vi "waitForIdleAndPrintTaskInfo.vi"(8 "error in (no error)":errorcluster, 9 "Timeout, ms (-1)":i32=-1, 10 "wait for ApplicationState (Idle)":i32(ring)=1448165379 items=["NotRunning"=1448165376, "Starting"=1448165377, "Dying"=1448165378, "Idle"=1448165379, "WorkInProgress"=1448165380], 11 "VGS_RemoteControlClient in":refnum<class "VGS_RemoteControlClient.lvclass">) -> (0 "error out":errorcluster, 3 "VGS_RemoteControlClient out":refnum<class "VGS_RemoteControlClient.lvclass">)   [LabVIEW 2022 SP3, in "LV_VGS.lvlib" / "VGS_RemoteControlClient.lvclass"]
uses:
  VGS_RemoteControlClient.lvclass
panel:
  # "< do not change default, please"
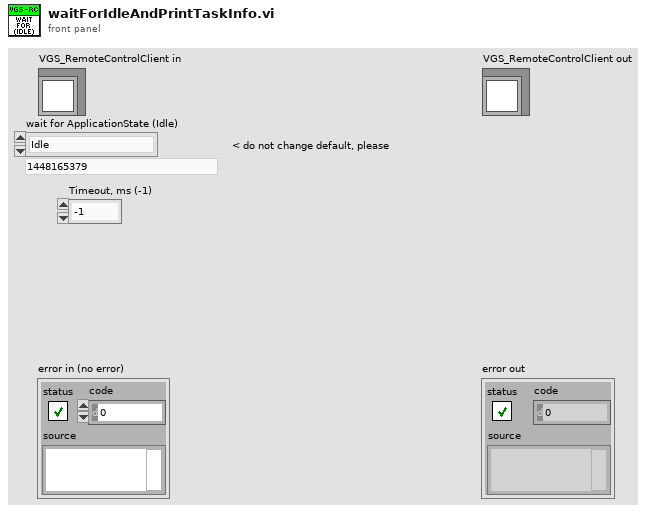
[diagram p1: front panel]
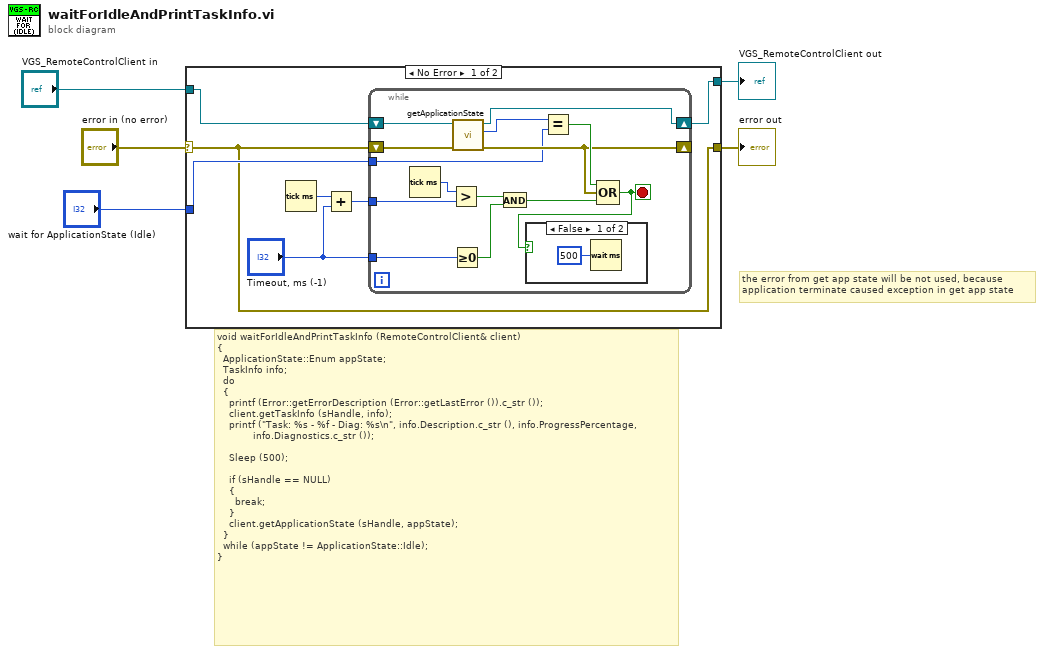
[diagram p0: block diagram]
diagram:
  # "the error from get app state will be not used, because\napplication terminate caused exception in get app state"
  # "void waitForIdleAndPrintTaskInfo (RemoteControlClient& client)\n{\n  ApplicationState::Enum appState;\n  TaskInfo info;\n  do\n  {\n    printf (Error::getErrorDescription (Error::getLastError ()).c_str ());\n    client.getTaskInfo (sHandle, info);\n    printf (\"Task: %s - %f - Diag: %s\\n\", info.Description.c_str (), info.ProgressPercentage,\n            info.Diagnostics.c_str ());\n\n    Sleep (500);\n\n    if (sHandle == NULL)\n    {\n      break;\n    }\n    client.getApplicationState (sHandle, appState);\n  }\n  while (appState != ApplicationState::Idle);\n}"
  n1 = case shown="No Error" "error in (no error)" {
    selector: "error in (no error)" -> [w6 w29]
    tunnel: [w6 w29] -> w4
    tunnel: [w11 w28] -> w2
    tunnel: "VGS_RemoteControlClient in" -> [w12 w28]
    tunnel: "wait for ApplicationState (Idle)" -> [w7 _]
    frame No Error {
      n2 = Tick Count (ms)() -> (millisecond timer value=w10:u32)
      n3 = Add(x=w10, y="Timeout, ms (-1)") -> (x+y=w9:u32)
      n4 = while {
        shift-right: [w26] -> w11
        shift-left: w12 -> [w13]
        shift-right: [w23] -> _
        shift-left: w6 -> [w14]
        tunnel: w9 -> [w21]
        tunnel: "Timeout, ms (-1)" -> [w19]
        tunnel: w7 -> [w16]
        stop <- w15 stop-if-true
        n5 = Tick Count (ms)() -> (millisecond timer value=w22:u32)
        n6 = Greater?(x=w22, y=w21) -> (0:w20:bool)
        n7 = Greater Or Equal To 0?(x=w19) -> (x >= 0?=w18:bool)
        n8 = call "getApplicationState.vi"("error in (no error)"=w14, "VGS_RemoteControlClient in"=w13) -> ("error out"=w23:errorcluster, "getApplicationState"=w25:i32, "VGS_RemoteControlClient out"=w26:refnum<class "VGS_RemoteControlClient.lvclass">)  [unwired: 7 in]
        n9 = And(x=w20, y=w18) -> (x .and. y?=w17:bool)
        n10 = Equal?(x=w25, y=w16) -> (x = y?=w24:bool)
        n11 = Compound Arithmetic op=OR(w24, w23, w17) -> (w15:bool)
        n12 = case shown="False" w15 {
          frame False {
            n13 = Wait (ms)(milliseconds to wait=u32 500) -> ()  [unwired: 1 out]
          }
          frame True {
          }
        }
      }
    }
    frame Error {
    }
  }
  "error out" <- w4
  "VGS_RemoteControlClient out" <- w2
